vi "RichToFlatcif_common_TimingStats.vi"(5 "OutputClusterType":T1, 11 "InputCluster":T2) -> (3 "OutputCluster":T1)   [LabVIEW 2021, in "CIF_PluginLoader_server.lvlib"]
uses:
  CIF_PluginLoader_server.lvlib
  cif_common_TimingStats.ctl
  cif_common_TimingStats_Flat.ctl
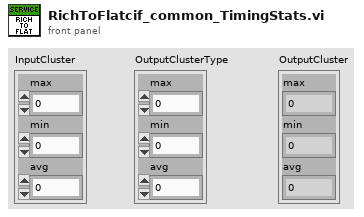
[diagram p1: front panel]
types:
  T1 = typedef "CIF_PluginLoader_server.lvlib/cif_common_TimingStats_Flat.ctl" = cluster{"max":i64, "min":i64, "avg":dbl}
  T2 = typedef "CIF_PluginLoader_server.lvlib/cif_common_TimingStats.ctl" = cluster{"max":i64, "min":i64, "avg":dbl}
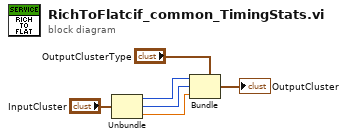
[diagram p0: block diagram]
diagram:
  n1 = Unbundle "Unbundle"("InputCluster") -> ("max"=w3:i64, "min"=w2:i64, "avg"=w1:dbl)
  n2 = Bundle "Bundle"(cluster="OutputClusterType", "max"=w3, "min"=w2, "avg"=w1) -> (→"OutputCluster":T1)
